vi "ADCP_get_parameter_details.vi"() -> ()   [LabVIEW 2017, in "ADCP.lvclass"]
uses:
  ADCP.lvclass
panel:
  in  "Parameter Name":string
  in  "error in (no error)":errorcluster
  in  "ADCP In":refnum<class "ADCP.lvclass">
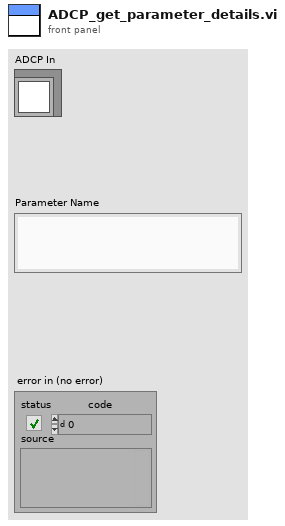
[diagram p1: front panel]
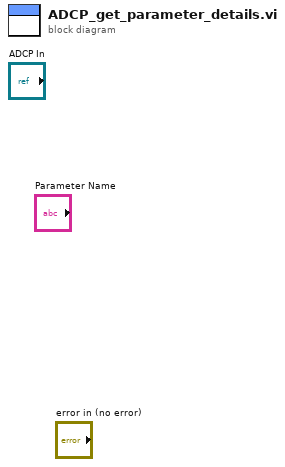
[diagram p0: block diagram]
diagram:
